vi "G#Debugger_RunMethod.vi"(0 "ClassPath":path, 1 "MethodName":string, 2 "ClassPrefix":string, 5 "error in (no error)":errorcluster, 6 "ControlValue":variant[](array[variant])) -> (15 "Error?":bool, 18 "ControlValue out":variant[](array[variant]), 19 "error out":errorcluster)   [LabVIEW 2017, in "G#Debugger.lvlib"]
uses:
  <vilib>/addons/_AddQ/G#Debugger/G#Debugger.lvlib
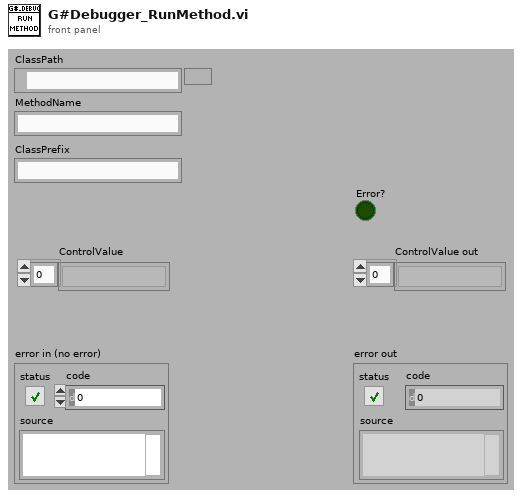
[diagram p1: front panel]
types:
  T1 = cluster{"ObjectName":string, "ObjectID":u32, "Users":i32, "Counter":bool, "AttributeRefs":u32[], "FullClassName":string, "ClassName":string, "Create method":enum16{"Create", "Create or look up existing", "Look up existing"}, "GenericDestructorExists":bool, "Owner":string}[]
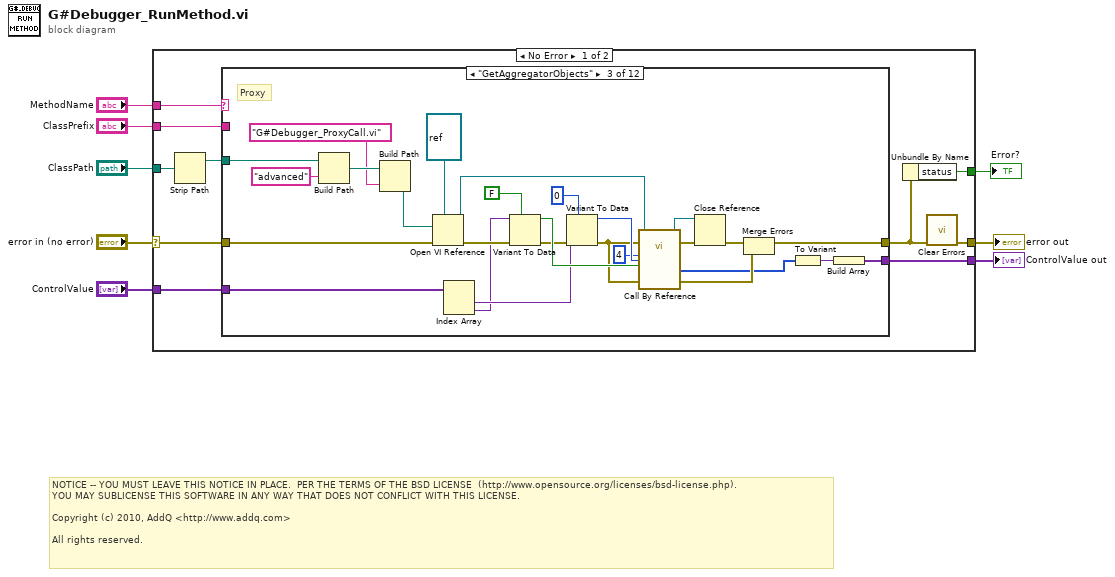
[diagram p0: block diagram]
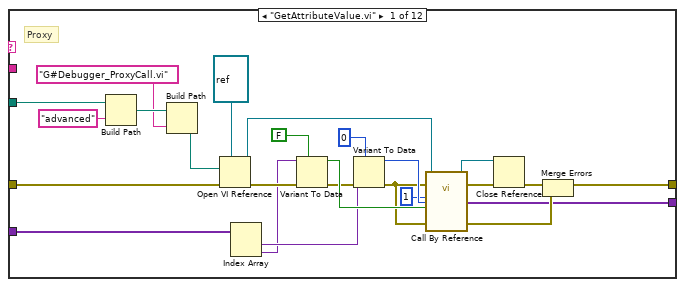
[diagram p2: hidden frame]
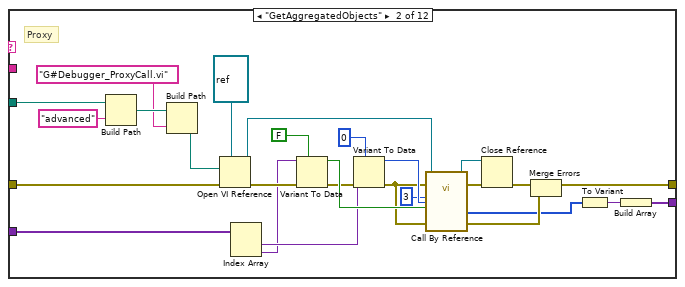
[diagram p3: hidden frame]
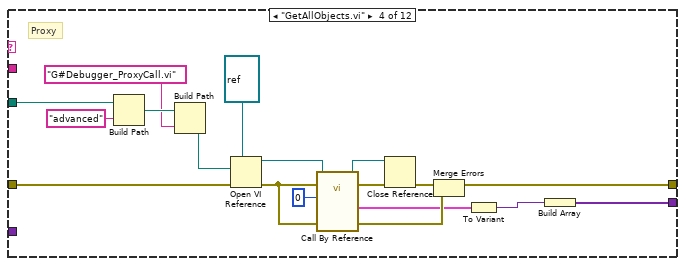
[diagram p4: hidden frame]
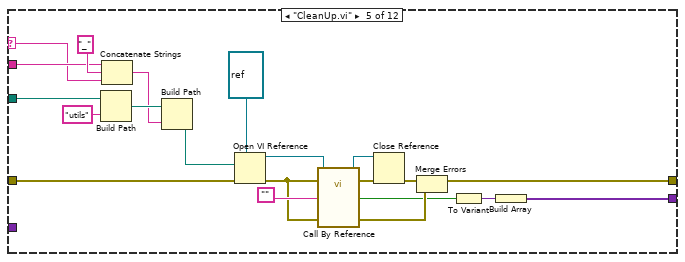
[diagram p5: hidden frame]
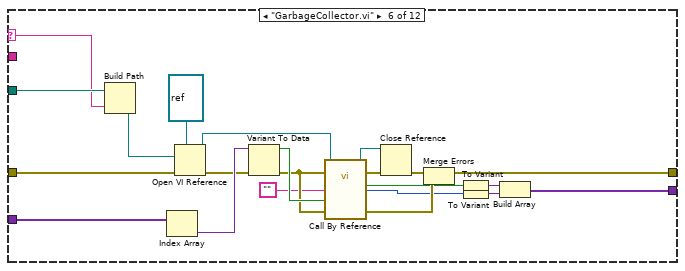
[diagram p6: hidden frame]
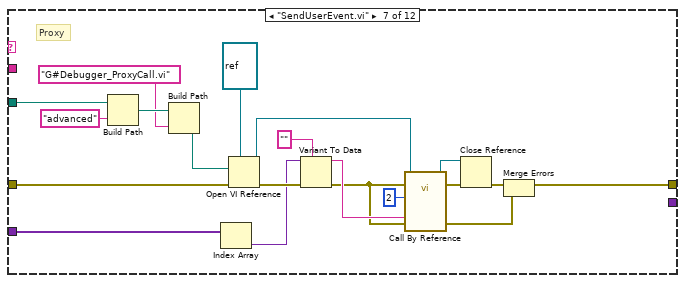
[diagram p7: hidden frame]
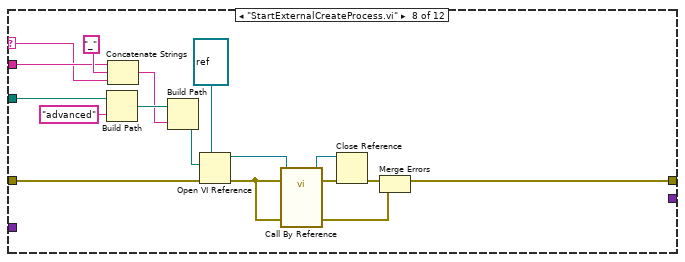
[diagram p8: hidden frame]
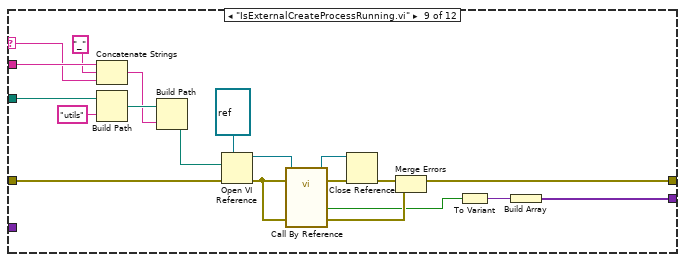
[diagram p9: hidden frame]
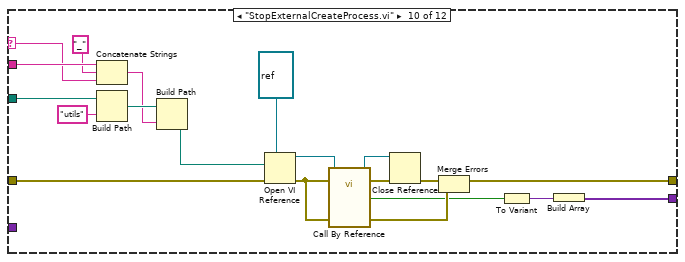
[diagram p10: hidden frame]
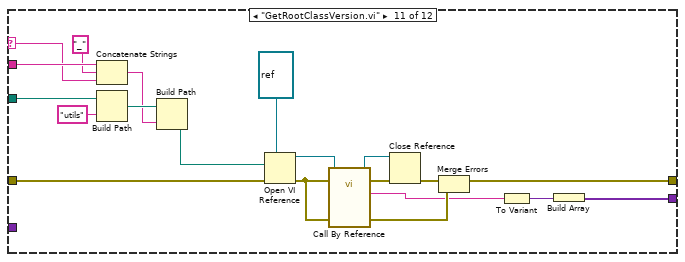
[diagram p11: hidden frame]
diagram:
  # "NOTICE -- YOU MUST LEAVE THIS NOTICE IN PLACE.  PER THE TERMS OF THE BSD LICENSE  (http://www.opensource.org/licenses/bsd-license.php).\nYOU MAY SUBLICENSE THIS SOFTWARE IN ANY WAY THAT DOES NOT CONFLICT WITH THIS LICENSE.\n\nCopyright (c) 2010, AddQ <http://www.addq.com>\n\nAll rights reserved."
  n1 = case shown="No Error" "error in (no error)" {
    selector: "error in (no error)" -> [w9 w257]
    tunnel: "ClassPath" -> [w18 _]
    tunnel: "ClassPrefix" -> [w10 _]
    tunnel: "MethodName" -> [w12 _]
    tunnel: [w15 w257] -> w5
    tunnel: "ControlValue" -> [w16 _]
    tunnel: [w17 _] -> w3
    tunnel: [w13 _] -> w1
    frame No Error {
      n2 = Strip Path(path=w18) -> (stripped path=w11:path)  [unwired: 1 out]
      n3 = case shown="\"GetAggregatorObjects\"" w12 {
        selector: w12 -> [_ _ _ _ w123 w137 _ w182 w203 w223 w243 _]
        tunnel: [w27 w44 w71 w104 w118 w147 _ _ w196 w216 w236 _] -> w17
        tunnel: w16 -> [w35 w62 w89 _ _ w150 w170 _ _ _ _ _]
        tunnel: [w39 w66 w93 w111 w132 w154 w174 w191 w211 w231 w251 w256] -> w14
        tunnel: w9 -> [w43 w70 w97 w115 w136 w158 w178 w195 w215 w235 w255 w256]
        tunnel: w11 -> [w20 w48 w75 w99 w122 w138 w160 w181 w206 w226 w246 _]
        tunnel: w10 -> [_ _ _ _ w124 _ _ w183 w205 w225 w245 _]
        frame "GetAttributeValue.vi" {
          # "Proxy"
          n4 = Build Path(base path=w20, name or relative path="advanced") -> (appended path=w23:path)
          n5 = Build Path(base path=w23, name or relative path="G#Debugger_ProxyCall.vi" ("string")) -> (appended path=w21:path)
          n6 = Open VI Reference(type specifier VI Refnum (for type only)=refnum<vi> refnum, vi path=w21, error in (no error)=w43) -> (vi reference=w41:refnum<vi>, error out=w29:errorcluster)  [unwired: 3 in]
          n7 = Index Array(array=w35) -> (element #1=w26:variant, element #2=w25:variant)  [unwired: 2 in]
          n8 = Variant To Data(error in=w29, type=FALSE, Variant=w25) -> (data=w31:bool, error out=w30:errorcluster)
          n9 = Variant To Data(error in=w30, type=u32 0 ("default (0 I32)"), Variant=w26) -> (data=w32:u32, error out=w28:errorcluster)
          n10 = call-by-ref "?"(reference=w41, error in=w28, "Method"=1 ("ObjectID"), "ObjectID"=w32, "ObjectAttributes (T)"=w31, 5:"error in (no error)"=w28) -> (reference out=w37:refnum<vi>, error out=w36:errorcluster, "Attributes"=w27:variant[], 19:"error out"=w38:errorcluster)  [unwired: 11 in, 3 out]
          n11 = Close Reference(reference=w37, error in (no error)=w36) -> (error out=w40:errorcluster)
          n12 = Merge Errors(w40, w38) -> (w39:errorcluster)
        }
        frame "GetAggregatedObjects" {
          # "Proxy"
          n13 = Build Path(base path=w48, name or relative path="advanced") -> (appended path=w51:path)
          n14 = Build Path(base path=w51, name or relative path="G#Debugger_ProxyCall.vi" ("string")) -> (appended path=w49:path)
          n15 = Open VI Reference(type specifier VI Refnum (for type only)=refnum<vi> refnum, vi path=w49, error in (no error)=w70) -> (vi reference=w68:refnum<vi>, error out=w56:errorcluster)  [unwired: 3 in]
          n16 = Index Array(array=w62) -> (element #1=w54:variant, element #2=w53:variant)  [unwired: 2 in]
          n17 = Variant To Data(error in=w56, type=FALSE, Variant=w53) -> (data=w58:bool, error out=w57:errorcluster)
          n18 = Variant To Data(error in=w57, type=u32 0 ("default (0 I32)"), Variant=w54) -> (data=w59:u32, error out=w55:errorcluster)
          n19 = call-by-ref "?"(reference=w68, error in=w55, "Method"=3 ("ObjectID"), "ObjectID"=w59, "ObjectAttributes (T)"=w58, 5:"error in (no error)"=w55) -> (reference out=w64:refnum<vi>, error out=w63:errorcluster, "ObjectIDs"=w45:u32[], 19:"error out"=w65:errorcluster)  [unwired: 11 in, 3 out]
          n20 = Close Reference(reference=w64, error in (no error)=w63) -> (error out=w67:errorcluster)
          n21 = Merge Errors(w67, w65) -> (w66:errorcluster)
          n22 = To Variant(anything=w45) -> (Variant=w46:variant)
          n23 = Build Array(w46) -> (w44:variant[])
        }
        frame "GetAggregatorObjects" {
          # "Proxy"
          n24 = Build Path(base path=w75, name or relative path="advanced") -> (appended path=w78:path)
          n25 = Build Path(base path=w78, name or relative path="G#Debugger_ProxyCall.vi" ("string")) -> (appended path=w76:path)
          n26 = Open VI Reference(type specifier VI Refnum (for type only)=refnum<vi> refnum, vi path=w76, error in (no error)=w97) -> (vi reference=w95:refnum<vi>, error out=w83:errorcluster)  [unwired: 3 in]
          n27 = Index Array(array=w89) -> (element #1=w81:variant, element #2=w80:variant)  [unwired: 2 in]
          n28 = Variant To Data(error in=w83, type=FALSE, Variant=w80) -> (data=w85:bool, error out=w84:errorcluster)
          n29 = Variant To Data(error in=w84, type=u32 0 ("default (0 I32)"), Variant=w81) -> (data=w86:u32, error out=w82:errorcluster)
          n30 = call-by-ref "?"(reference=w95, error in=w82, "Method"=4 ("ObjectID"), "ObjectID"=w86, "ObjectAttributes (T)"=w85, 5:"error in (no error)"=w82) -> (reference out=w91:refnum<vi>, error out=w90:errorcluster, "ObjectIDs"=w72:u32[], 19:"error out"=w92:errorcluster)  [unwired: 11 in, 3 out]
          n31 = Close Reference(reference=w91, error in (no error)=w90) -> (error out=w94:errorcluster)
          n32 = Merge Errors(w94, w92) -> (w93:errorcluster)
          n33 = To Variant(anything=w72) -> (Variant=w73:variant)
          n34 = Build Array(w73) -> (w71:variant[])
        }
        frame "GetAllObjects.vi" {
          # "Proxy"
          n35 = Build Path(base path=w99, name or relative path="advanced") -> (appended path=w102:path)
          n36 = Build Path(base path=w102, name or relative path="G#Debugger_ProxyCall.vi" ("string")) -> (appended path=w98:path)
          n37 = Open VI Reference(type specifier VI Refnum (for type only)=refnum<vi> refnum, vi path=w98, error in (no error)=w115) -> (vi reference=w113:refnum<vi>, error out=w106:errorcluster)  [unwired: 3 in]
          n38 = call-by-ref "?"(reference=w113, error in=w106, "Method"=0, 5:"error in (no error)"=w106) -> (reference out=w109:refnum<vi>, error out=w108:errorcluster, "AllObjects"=w107:T1, 19:"error out"=w110:errorcluster)  [unwired: 13 in, 3 out]
          n39 = Close Reference(reference=w109, error in (no error)=w108) -> (error out=w112:errorcluster)
          n40 = Merge Errors(w112, w110) -> (w111:errorcluster)
          n41 = To Variant(anything=w107) -> (Variant=w105:variant)
          n42 = Build Array(w105) -> (w104:variant[])
        }
        frame "CleanUp.vi" {
          n43 = Build Path(base path=w122, name or relative path="utils") -> (appended path=w127:path)
          n44 = Concatenate Strings(w124, "_" ("string"), w123) -> (w125:string)
          n45 = Build Path(base path=w127, name or relative path=w125) -> (appended path=w121:path)
          n46 = Open VI Reference(type specifier VI Refnum (for type only)=refnum<vi> refnum, vi path=w121, error in (no error)=w136) -> (vi reference=w134:refnum<vi>, error out=w116:errorcluster)  [unwired: 3 in]
          n47 = call-by-ref "?"(reference=w134, error in=w116, "full class name (\"\")"="", 5:"error in (no error)"=w116) -> (reference out=w130:refnum<vi>, error out=w129:errorcluster, "any dead objects?"=w120:bool, 19:"error out"=w131:errorcluster)  [unwired: 16 in]
          n48 = Close Reference(reference=w130, error in (no error)=w129) -> (error out=w133:errorcluster)
          n49 = Merge Errors(w133, w131) -> (w132:errorcluster)
          n50 = To Variant(anything=w120) -> (Variant=w119:variant)
          n51 = Build Array(w119) -> (w118:variant[])
        }
        frame "GarbageCollector.vi" {
          n52 = Build Path(base path=w138, name or relative path=w137) -> (appended path=w149:path)
          n53 = Index Array(array=w150) -> (element=w141:variant)  [unwired: 1 in]
          n54 = Open VI Reference(type specifier VI Refnum (for type only)=refnum<vi> refnum, vi path=w149, error in (no error)=w158) -> (vi reference=w156:refnum<vi>, error out=w140:errorcluster)  [unwired: 3 in]
          n55 = Variant To Data(error in=w140, Variant=w141) -> (data=w143:bool, error out=w142:errorcluster)  [unwired: 1 in]
          n56 = call-by-ref "?"(reference=w156, error in=w142, "full class name"="", "only from same owner as caller? (T)"=w143, 5:"error in (no error)"=w142) -> (reference out=w152:refnum<vi>, error out=w151:errorcluster, "OK"=w144:bool, "# of objects killed"=w146:i32, 19:"error out"=w153:errorcluster)  [unwired: 14 in]
          n57 = Close Reference(reference=w152, error in (no error)=w151) -> (error out=w155:errorcluster)
          n58 = Merge Errors(w155, w153) -> (w154:errorcluster)
          n59 = To Variant(anything=w144) -> (Variant=w148:variant)
          n60 = To Variant(anything=w146) -> (Variant=w145:variant)
          n61 = Build Array(w148, w145) -> (w147:variant[])
        }
        frame "SendUserEvent.vi" {
          # "Proxy"
          n62 = Build Path(base path=w160, name or relative path="advanced") -> (appended path=w163:path)
          n63 = Build Path(base path=w163, name or relative path="G#Debugger_ProxyCall.vi" ("string")) -> (appended path=w159:path)
          n64 = Index Array(array=w170) -> (element=w166:variant)  [unwired: 1 in]
          n65 = Open VI Reference(type specifier VI Refnum (for type only)=refnum<vi> refnum, vi path=w159, error in (no error)=w178) -> (vi reference=w176:refnum<vi>, error out=w167:errorcluster)  [unwired: 3 in]
          n66 = Variant To Data(error in=w167, type="", Variant=w166) -> (data=w169:string, error out=w165:errorcluster)
          n67 = call-by-ref "?"(reference=w176, error in=w165, "Method"=2, "Text"=w169, 5:"error in (no error)"=w165) -> (reference out=w172:refnum<vi>, error out=w171:errorcluster, 19:"error out"=w173:errorcluster)  [unwired: 12 in, 4 out]
          n68 = Close Reference(reference=w172, error in (no error)=w171) -> (error out=w175:errorcluster)
          n69 = Merge Errors(w175, w173) -> (w174:errorcluster)
        }
        frame "StartExternalCreateProcess.vi" {
          n70 = Build Path(base path=w181, name or relative path="advanced") -> (appended path=w186:path)
          n71 = Concatenate Strings(w183, "_" ("string"), w182) -> (w184:string)
          n72 = Build Path(base path=w186, name or relative path=w184) -> (appended path=w180:path)
          n73 = Open VI Reference(type specifier VI Refnum (for type only)=refnum<vi> refnum, vi path=w180, error in (no error)=w195) -> (vi reference=w193:refnum<vi>, error out=w179:errorcluster)  [unwired: 3 in]
          n74 = call-by-ref "?"(reference=w193, error in=w179, 5:"error in (no error)"=w179) -> (reference out=w189:refnum<vi>, error out=w188:errorcluster, 19:"error out"=w190:errorcluster)  [unwired: 18 in]
          n75 = Close Reference(reference=w189, error in (no error)=w188) -> (error out=w192:errorcluster)
          n76 = Merge Errors(w192, w190) -> (w191:errorcluster)
        }
        frame "IsExternalCreateProcessRunning.vi" {
          n77 = Concatenate Strings(w205, "_" ("string"), w203) -> (w200:string)
          n78 = Build Path(base path=w206, name or relative path="utils") -> (appended path=w202:path)
          n79 = Build Path(base path=w202, name or relative path=w200) -> (appended path=w199:path)
          n80 = Open VI Reference(type specifier VI Refnum (for type only)=refnum<vi> refnum, vi path=w199, error in (no error)=w215) -> (vi reference=w213:refnum<vi>, error out=w207:errorcluster)  [unwired: 3 in]
          n81 = call-by-ref "?"(reference=w213, error in=w207, 5:"error in (no error)"=w207) -> (reference out=w209:refnum<vi>, error out=w208:errorcluster, "external create process running?"=w198:bool, 19:"error out"=w210:errorcluster)  [unwired: 15 in, 2 out]
          n82 = Close Reference(reference=w209, error in (no error)=w208) -> (error out=w212:errorcluster)
          n83 = Merge Errors(w212, w210) -> (w211:errorcluster)
          n84 = To Variant(anything=w198) -> (Variant=w197:variant)
          n85 = Build Array(w197) -> (w196:variant[])
        }
        frame "StopExternalCreateProcess.vi" {
          n86 = Concatenate Strings(w225, "_" ("string"), w223) -> (w220:string)
          n87 = Build Path(base path=w226, name or relative path="utils") -> (appended path=w222:path)
          n88 = Build Path(base path=w222, name or relative path=w220) -> (appended path=w219:path)
          n89 = Open VI Reference(type specifier VI Refnum (for type only)=refnum<vi> refnum, vi path=w219, error in (no error)=w235) -> (vi reference=w233:refnum<vi>, error out=w227:errorcluster)  [unwired: 3 in]
          n90 = call-by-ref "?"(reference=w233, error in=w227, 5:"error in (no error)"=w227) -> (reference out=w229:refnum<vi>, error out=w228:errorcluster, "stopped?"=w218:bool, 19:"error out"=w230:errorcluster)  [unwired: 17 in]
          n91 = Close Reference(reference=w229, error in (no error)=w228) -> (error out=w232:errorcluster)
          n92 = Merge Errors(w232, w230) -> (w231:errorcluster)
          n93 = To Variant(anything=w218) -> (Variant=w217:variant)
          n94 = Build Array(w217) -> (w216:variant[])
        }
        frame "GetRootClassVersion.vi" {
          n95 = Concatenate Strings(w245, "_" ("string"), w243) -> (w240:string)
          n96 = Build Path(base path=w246, name or relative path="utils") -> (appended path=w242:path)
          n97 = Build Path(base path=w242, name or relative path=w240) -> (appended path=w239:path)
          n98 = Open VI Reference(type specifier VI Refnum (for type only)=refnum<vi> refnum, vi path=w239, error in (no error)=w255) -> (vi reference=w253:refnum<vi>, error out=w247:errorcluster)  [unwired: 3 in]
          n99 = call-by-ref "?"(reference=w253, error in=w247, 5:"error in (no error)"=w247) -> (reference out=w249:refnum<vi>, error out=w248:errorcluster, "version"=w238:string, 19:"error out"=w250:errorcluster)  [unwired: 17 in]
          n100 = Close Reference(reference=w249, error in (no error)=w248) -> (error out=w252:errorcluster)
          n101 = Merge Errors(w252, w250) -> (w251:errorcluster)
          n102 = To Variant(anything=w238) -> (Variant=w237:variant)
          n103 = Build Array(w237) -> (w236:variant[])
        }
        frame Default {
        }
      }
      n104 = Unbundle By Name(w14) -> ("status"=w13:bool)
      n105 = call <vilib>:"Clear Errors.vi"("error in (no error)"=w14) -> ("error out"=w15:errorcluster)  [unwired: 5 in, 1 out]
    }
    frame Error {
    }
  }
  "error out" <- w5
  "ControlValue out" <- w3
  "Error?" <- w1
